vi "判定胜负.vi"(0 "当前棋盘状态":i32[][](array[numeric]), 7 "行":sgl, 9 "列":i16) -> (4 "当前棋盘状态":i32[][](array[numeric]), 8 "行":sgl, 10 "列":i16, 13 "此局结束?":bool, 14 "白子胜?":bool, 15 "黑子胜?":bool)   [LabVIEW 2018]
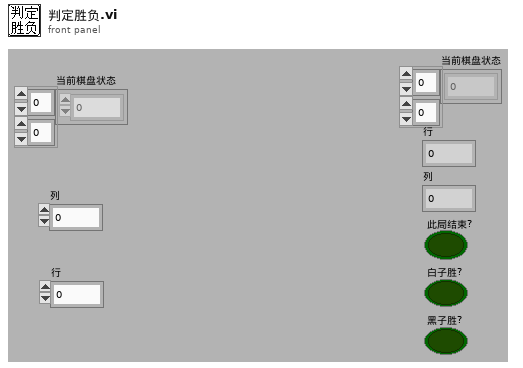
[diagram p1: front panel]
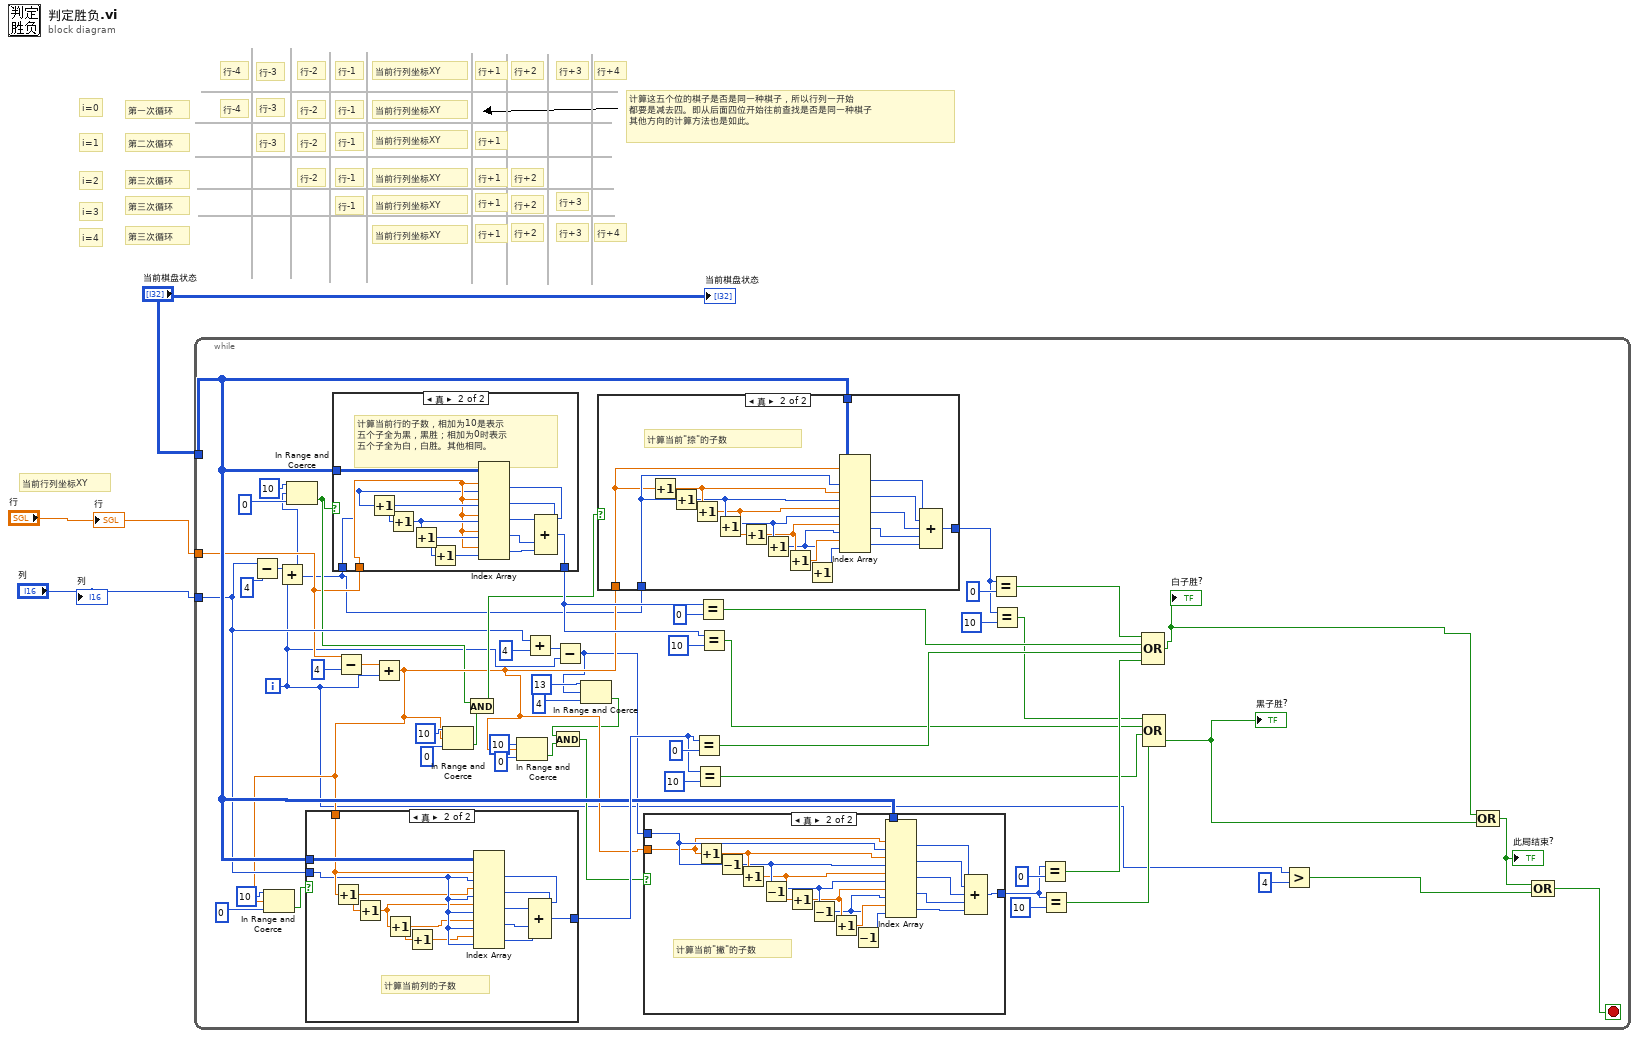
[diagram p0: block diagram]
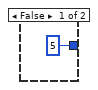
[diagram p2: hidden frame]
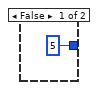
[diagram p3: hidden frame]
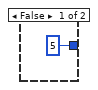
[diagram p4: hidden frame]
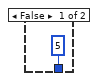
[diagram p5: hidden frame]
diagram:
  # "当前行列坐标XY"
  # "行+4"
  # "行+3"
  # "行+2"
  # "行+1"
  # "当前行列坐标XY"
  # "i=4"
  # "i=3"
  # "i=2"
  # "i=1"
  # "i=0"
  # "第三次循环"
  # "行+3"
  # "行+2"
  # "行+1"
  # "当前行列坐标XY"
  # "行-1"
  # "第三次循环"
  # "行+2"
  # "行+1"
  # "当前行列坐标XY"
  # "行-1"
  # "行-2"
  # "第三次循环"
  # "行+1"
  # "当前行列坐标XY"
  # "行-1"
  # "行-2"
  # "行-3"
  # "第二次循环"
  # "计算这五个位的棋子是否是同一种棋子，所以行列一开始\n都要是减去四。即从后面四位开始往前查找是否是同一种棋子\n其他方向的计算方法也是如此。"
  # "当前行列坐标XY"
  # "行-1"
  # "行-2"
  # "行-3"
  # "行-4"
  # "第一次循环"
  # "行-4"
  # "行-3"
  # "行-2"
  # "行-1"
  # "行+4"
  # "行+3"
  # "行+2"
  # "行+1"
  # "当前行列坐标XY"
  n1 = while {
    tunnel: "行" -> [w20]
    tunnel: "当前棋盘状态" -> [w46]
    tunnel: "列" -> [w38]
    i -> [w9]
    stop <- w6 stop-if-true
    n2 = Subtract(x=w38, y=u8 4) -> (x-y=w59:i16)
    n3 = Add(x=w59, y=w9) -> (x+y=w19:i32)
    n4 = In Range and Coerce(upper limit=u8 10, x=w19, lower limit=u8 0) -> (In Range?=w26:bool)  [unwired: 1 out]
    n5 = case shown="真" w26 {
      tunnel: w46 -> [_ w114]
      tunnel: w20 -> [_ w112]
      tunnel: w19 -> [_ w111]
      tunnel: [5 w113] -> w53
      frame False {
      }
      frame True {
        # "计算当前行的子数，相加为10是表示\n五个子全为黑，黑胜；相加为0时表示\n五个子全为白，白胜。其他相同。"
        n6 = Increment(x=w111) -> (x+1=w123:i32)
        n7 = Increment(x=w123) -> (x+1=w122:i32)
        n8 = Increment(x=w122) -> (x+1=w120:i32)
        n9 = Increment(x=w120) -> (x+1=w121:i32)
        n10 = Index Array(array=w114, index (row) #1=w112, index (col) #1=w111, index (row) #2=w112, index (col) #2=w123, index (row) #3=w112, index (col) #3=w122, index (row) #4=w112, index (col) #4=w120, index (row) #5=w112, index (col) #5=w121) -> (element #1=w119:i32, element #2=w118:i32, element #3=w117:i32, element #4=w116:i32, element #5=w115:i32)
        n11 = Compound Arithmetic op=ADD(w119, w118, w117, w116, w115) -> (w113:i32)
      }
    }
    n12 = Subtract(x=w20, y=u8 4) -> (x-y=w56:sgl)
    n13 = Add(x=w56, y=w9) -> (x+y=w28:sgl)
    n14 = In Range and Coerce(upper limit=u8 10, x=w28, lower limit=u8 0) -> (In Range?=w29:bool)  [unwired: 1 out]
    n15 = case shown="真" w29 {
      tunnel: w46 -> [_ w104]
      tunnel: w38 -> [_ w101]
      tunnel: w28 -> [_ w102]
      tunnel: [5 w103] -> w47
      frame False {
      }
      frame True {
        # "计算当前列的子数"
        n16 = Increment(x=w102) -> (x+1=w97:sgl)
        n17 = Increment(x=w97) -> (x+1=w98:sgl)
        n18 = Increment(x=w98) -> (x+1=w99:sgl)
        n19 = Increment(x=w99) -> (x+1=w100:sgl)
        n20 = Index Array(array=w104, index (row) #1=w102, index (col) #1=w101, index (row) #2=w97, index (col) #2=w101, index (row) #3=w98, index (col) #3=w101, index (row) #4=w99, index (col) #4=w101, index (row) #5=w100, index (col) #5=w101) -> (element #1=w105:i32, element #2=w106:i32, element #3=w107:i32, element #4=w108:i32, element #5=w109:i32)
        n21 = Compound Arithmetic op=ADD(w105, w106, w107, w108, w109) -> (w103:i32)
      }
    }
    n22 = In Range and Coerce(upper limit=u8 10, x=w28, lower limit=u8 0) -> (In Range?=w37:bool)  [unwired: 1 out]
    n23 = And(x=w26, y=w37) -> (x .and. y?=w42:bool)
    n24 = In Range and Coerce(upper limit=u8 10, x=w28, lower limit=u8 0) -> (In Range?=w32:bool)  [unwired: 1 out]
    n25 = Add(x=w38, y=u8 4) -> (x+y=w39:i16)
    n26 = Subtract(x=w39, y=w9) -> (x-y=w21:i32)
    n27 = In Range and Coerce(upper limit=u8 13, x=w21, lower limit=u8 4) -> (In Range?=w22:bool)  [unwired: 1 out]
    n28 = And(x=w22, y=w32) -> (x .and. y?=w41:bool)
    n29 = case shown="真" w42 {
      tunnel: w46 -> [_ w90]
      tunnel: [5 w81] -> w50
      tunnel: w19 -> [_ w80]
      tunnel: w28 -> [_ w79]
      frame False {
      }
      frame True {
        # "计算当前\"捺\"的子数"
        n30 = Increment(x=w79) -> (x+1=w87:sgl)
        n31 = Increment(x=w80) -> (x+1=w86:i32)
        n32 = Increment(x=w87) -> (x+1=w85:sgl)
        n33 = Increment(x=w86) -> (x+1=w84:i32)
        n34 = Increment(x=w85) -> (x+1=w83:sgl)
        n35 = Increment(x=w84) -> (x+1=w82:i32)
        n36 = Increment(x=w83) -> (x+1=w89:sgl)
        n37 = Increment(x=w82) -> (x+1=w88:i32)
        n38 = Index Array(array=w90, index (row) #1=w79, index (col) #1=w80, index (row) #2=w87, index (col) #2=w86, index (row) #3=w85, index (col) #3=w84, index (row) #4=w83, index (col) #4=w82, index (row) #5=w89, index (col) #5=w88) -> (element #1=w91:i32, element #2=w92:i32, element #3=w93:i32, element #4=w94:i32, element #5=w95:i32)
        n39 = Compound Arithmetic op=ADD(w91, w92, w93, w94, w95) -> (w81:i32)
      }
    }
    n40 = case shown="真" w41 {
      tunnel: w46 -> [_ w72]
      tunnel: [5 w63] -> w43
      tunnel: w21 -> [_ w62]
      tunnel: w28 -> [_ w61]
      frame False {
      }
      frame True {
        # "计算当前\"撇\"的子数"
        n41 = Increment(x=w61) -> (x+1=w69:sgl)
        n42 = Decrement(x=w62) -> (x-1=w68:i32)
        n43 = Increment(x=w69) -> (x+1=w67:sgl)
        n44 = Decrement(x=w68) -> (x-1=w66:i32)
        n45 = Increment(x=w67) -> (x+1=w65:sgl)
        n46 = Decrement(x=w66) -> (x-1=w64:i32)
        n47 = Increment(x=w65) -> (x+1=w71:sgl)
        n48 = Decrement(x=w64) -> (x-1=w70:i32)
        n49 = Index Array(array=w72, index (row) #1=w61, index (col) #1=w62, index (row) #2=w69, index (col) #2=w68, index (row) #3=w67, index (col) #3=w66, index (row) #4=w65, index (col) #4=w64, index (row) #5=w71, index (col) #5=w70) -> (element #1=w73:i32, element #2=w74:i32, element #3=w75:i32, element #4=w76:i32, element #5=w77:i32)
        n50 = Compound Arithmetic op=ADD(w73, w74, w75, w76, w77) -> (w63:i32)
      }
    }
    n51 = Equal?(x=w47, y=0) -> (x = y?=w16:bool)
    n52 = Equal?(x=w47, y=10) -> (x = y?=w12:bool)
    n53 = Equal?(x=w53, y=0) -> (x = y?=w17:bool)
    n54 = Equal?(x=w53, y=10) -> (x = y?=w13:bool)
    n55 = Equal?(x=w50, y=0) -> (x = y?=w18:bool)
    n56 = Equal?(x=w50, y=10) -> (x = y?=w14:bool)
    n57 = Equal?(x=w43, y=0) -> (x = y?=w15:bool)
    n58 = Equal?(x=w43, y=10) -> (x = y?=w11:bool)
    n59 = Compound Arithmetic op=OR(w18, w17, w16, w15) -> (w5:bool)
    "白子胜?" <- w5
    n60 = Compound Arithmetic op=OR(w14, w13, w12, w11) -> (w4:bool)
    "黑子胜?" <- w4
    n61 = Greater?(x=w9, y=u8 4) -> (0:w7:bool)
    n62 = Compound Arithmetic op=OR(w5, w4) -> (w8:bool)
    "此局结束?" <- w8
    n63 = Compound Arithmetic op=OR(w8, w7) -> (w6:bool)
  }
  "当前棋盘状态" <- "当前棋盘状态"
  "行" <- "行"
  "列" <- "列"
